vi "Configure test.vi"(6 "Assert VI Path":path, 7 "Existing Queue Elements":string, 8 "error in (no error)":errorcluster, 11 "Basic Int GTLT in":refnum<class "Int GTLT.lvclass">) -> (0 "error out":errorcluster, 3 "Basic Int GTLT out":refnum<class "Int GTLT.lvclass">)   [LabVIEW 2018, in "Int GTLT.lvclass"]
uses:
  Int GTLT.lvclass
  84be06c2-4681-49e4-80e3-b68ac4b8209a.vi
  <vilib>/JDP Science/JSONtext/Find Item.vi
  84be06c2-4681-49e4-80e3-b68ac4b8209a.vi/a64efc3d-73a3-4adc-ae0f-21d269176d8f.vi
  84be06c2-4681-49e4-80e3-b68ac4b8209a.vi/a3189823-b2ea-4b28-b825-92bdac172e9f.vi
  <vilib>/JDP Science/JSONtext/String Subset.vi
  Test Class String IDs.vi
  <vilib>/JDP Science/JSONtext/Parsing/Parse Full Path or Item Name.vi
  <vilib>/JDP Science/JSONtext/Offset/Find Item Locations by Path.vi
  <vilib>/JDP Science/JSONtext/JSON text to Variant.vi
  <vilib>/JDP Science/JSONtext/Variant to JSON Text.vi
  <vilib>/JDP Science/JSONtext/Set Item.vi
  Integer.lvclass
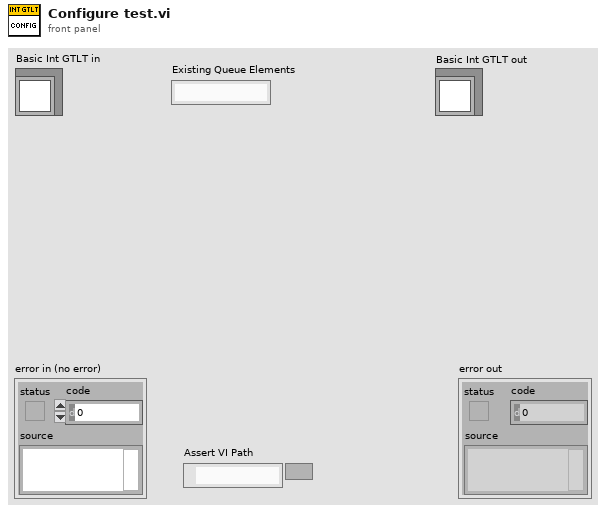
[diagram p1: front panel]
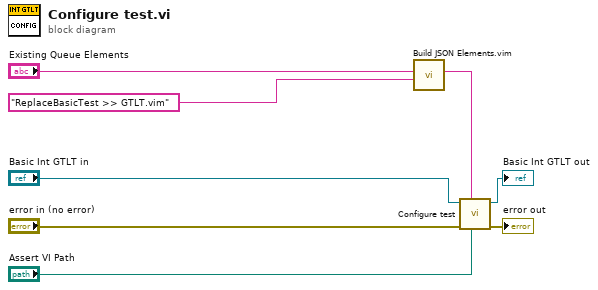
[diagram p0: block diagram]
diagram:
  n1 = call "Build JSON Elements.vim"("Append Element(s)"="ReplaceBasicTest >> GTLT.vim", "JSON Elements in ({})"="Existing Queue Elements") -> ("JSON Elements out"=w1:string)  [unwired: 9 in]
  n2 = call-parent "Configure test.vi"("Assert VI Path"="Assert VI Path", "Existing Queue Elements"=w1, "error in (no error)"="error in (no error)", "Basic Integer in"="Basic Int GTLT in") -> ("error out"=→"error out":errorcluster, "Basic Integer out"=→"Basic Int GTLT out":refnum<class "Int GTLT.lvclass">)  [unwired: 6 in]
